vi "Configure Scale.vi"(5 "Scaling Function (0: dB)":i32(ring) items=["dB", "dBM"], 6 "Enable Scaling (F: Disable)":bool, 7 "Auto Reference (T: Enable)":bool=TRUE, 8 "error in (no error)":errorcluster, 9 "Reference Resistance (600: 600 ohm)":i32(ring)=600 items=["50"=50, "75"=75, "93"=93, "110"=110, "124"=124, "125"=125, "135"=135, "150"=150, "250"=250, "300"=300, "500"=500, "600"=600, "800"=800, "900"=900, "1000"=1000, "1200"=1200, "8000"=8000], 10 "Relative Value (0 dBm)":dbl, 11 "VISA resource name":refnum<visa-resource-name>) -> (0 "error out":errorcluster, 3 "VISA resource name out":refnum<visa-resource-name>)   [LabVIEW 2013, in "Agilent 3446X Series.lvlib"]
doc: "Configures scale settings.\n\n<B>Note(s):</B>\nThis VI applies only to ACV and DCV measurement functions."
uses:
  Agilent 3446X Series.lvlib
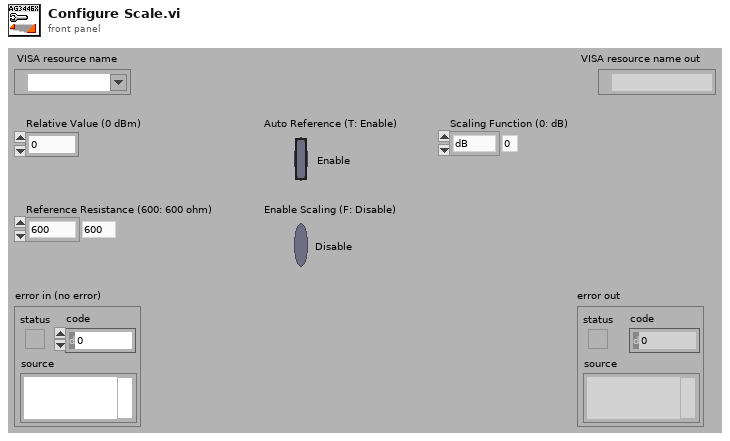
[diagram p1: front panel]
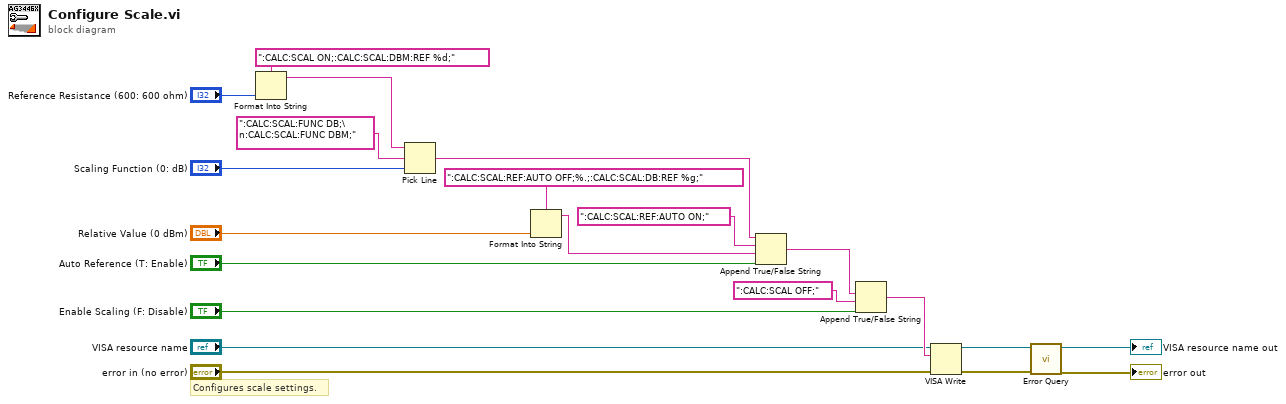
[diagram p0: block diagram]
diagram:
  # "Configures scale settings."
  n1 = Format Into String(format string=":CALC:SCAL ON;:CALC:SCAL:DBM:REF %d;", "Reference Resistance (600: 600 ohm)") -> (resulting string=w4:string)  [unwired: 2 in, 1 out]
  n2 = Pick Line(string ("")=w4, multi-line string=":CALC:SCAL:FUNC DB;\n:CALC:SCAL:FUNC DBM;", line index="Scaling Function (0: dB)") -> (output string=w1:string)
  n3 = Format Into String(format string=":CALC:SCAL:REF:AUTO OFF;%.;:CALC:SCAL:DB:REF %g;", "Relative Value (0 dBm)") -> (resulting string=w5:string)  [unwired: 2 in, 1 out]
  n4 = Append True/False String(1:"Auto Reference (T: Enable)", 2:w5, 3:":CALC:SCAL:REF:AUTO ON;", 4:w1) -> (0:w3:string)
  n5 = Append True/False String(1:"Enable Scaling (F: Disable)", 2:":CALC:SCAL OFF;", 3:w3) -> (0:w12:string)  [unwired: 1 out]
  n6 = VISA Write(VISA resource name="VISA resource name", write buffer=w12, error in (no error)="error in (no error)") -> (VISA resource name out=w9:refnum<visa-resource-name>, error out=w8:errorcluster)  [unwired: 1 out]
  n7 = call "Error Query.vi"("error in (no error)"=w8, "VISA resource name"=w9) -> ("error out"=→"error out":errorcluster, "VISA resource name out"=→"VISA resource name out":refnum<visa-resource-name>)  [unwired: 8 out]
